vi "Set Values From HovaCAL Input.vi"(8 "error in (no error)":errorcluster caption="Fehler (Eingang, kein Fehler)") -> (0 "error out":errorcluster caption="Fehler (Ausgang)", 1 "HovaCAL Temperature":dbl[](array[numeric]) caption="Temp Setpoint" format="%.2f", 2 "SetPumpMode-Cluster":T4(array[cluster]) {"concentratio mode" items=["water", "reagent"]; "Reagent" items=["HCl", "HF", "NH3", "HG", "PPM", "ORGANIC"]}, 3 "Cluster.PumpModeGeneral":T8 caption="Pump Mode" {"dry mode" items=["wet", "dry"]; "control mode" items=["static", "pid"]}, 4 "Pump Concentrations-Cluster":T1[](array[typedef]) caption="Pump Setpoint", 5 "Set Values Cluster":T5(array[cluster]) caption="MFC Setpoints" {"output concentration setpoint" format="%.2f"; "input concentration setpoint" format="%.2f"}, 6 "Flow Input Cluster":cluster{"total flow setpoint":dbl} caption="Flow Setpoint" {"total flow setpoint" format="%.2f"}, 7 "Limits Cluster":cluster{"flow":dbl[], "temp":dbl[]} caption="Limits", 11 "SetPumpMode":cluster{"run":bool} caption="Pump")   [LabVIEW 2020, in "Linearisierung v2.lvlib" / "Gasteiler.lvlib" / "HovaCAL_Interface.lvlib" / "Kommunikation.lvlib"]
uses:
  Kommunikation.lvlib
  Controls/Pump Dry Mode.ctl
  Controls/Pump Control Mode.ctl
  Controls/Pump Concentration Mode.ctl
  Controls/Reagent.ctl
  Controls/Pump Concentration.ctl
  Aktion_FGV_HovaCAL_Interface_GetData.ctl
  Controls/Controls.lvlib
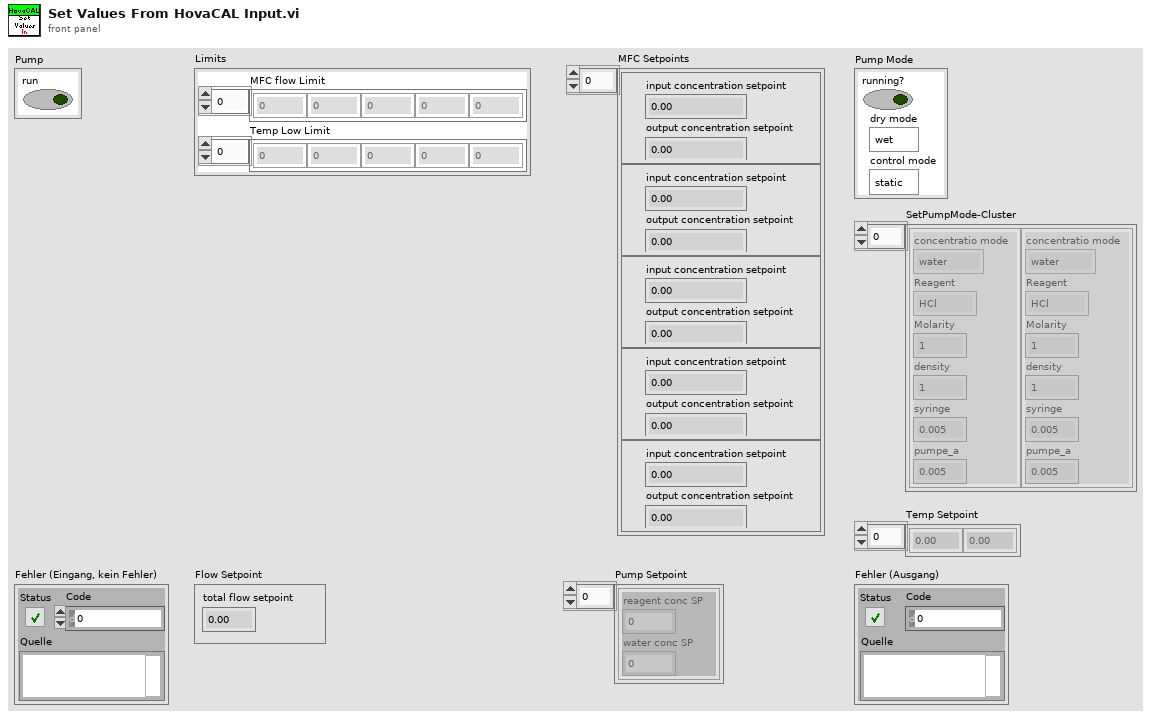
[diagram p1: front panel]
types:
  T1 = typedef "Linearisierung v2.lvlib/Gasteiler.lvlib/HovaCAL_Interface.lvlib/Controls.lvlib/Pump Concentration.ctl" = cluster{"reagent conc SP":dbl, "water conc SP":dbl}
  T2 = typedef "Linearisierung v2.lvlib/Gasteiler.lvlib/HovaCAL_Interface.lvlib/Controls.lvlib/Pump Concentration Mode.ctl" = i32
  T3 = typedef "Linearisierung v2.lvlib/Gasteiler.lvlib/HovaCAL_Interface.lvlib/Controls.lvlib/Reagent.ctl" = i32
  T4 = cluster{"concentratio mode":T2, "Reagent":T3, "Molarity":dbl, "density":dbl, "syringe":dbl, "pumpe_a":dbl}[]
  T5 = cluster{"input concentration setpoint":dbl, "output concentration setpoint":dbl}[]
  T6 = typedef "Linearisierung v2.lvlib/Gasteiler.lvlib/HovaCAL_Interface.lvlib/Controls.lvlib/Pump Dry Mode.ctl" = i32
  T7 = typedef "Linearisierung v2.lvlib/Gasteiler.lvlib/HovaCAL_Interface.lvlib/Controls.lvlib/Pump Control Mode.ctl" = u32
  T8 = cluster{"running?":bool, "dry mode":T6, "control mode":T7}
  T9 = cluster{"reagent conc SP":dbl, "water conc SP":dbl}
  T10 = cluster{"concentratio mode":T2, "Reagent":T3, "Molarity":dbl, "density":dbl, "syringe":dbl, "pumpe_a":dbl}
  T11 = cluster{"input concentration setpoint":dbl, "output concentration setpoint":dbl}
  T12 = typedef "Linearisierung v2.lvlib/Gasteiler.lvlib/HovaCAL_Interface.lvlib/Kommunikation.lvlib/Aktion_FGV_HovaCAL_Interface_GetData.ctl" = enum16{"lesen", "SystemInfo", "MFC Info", "actual Values", "Limits", "first contact", "reset after read"}
  T13 = cluster{"Input Concentrations (Ausgang)":cluster{"input concentration setpoint":dbl, "output concentration setpoint":dbl, "output concentration":dbl, "output concentration dry":dbl}[], "Cluster":cluster{"Temp Cluster":cluster{"temp SP":dbl, "temp":dbl, "humidity":dbl}[], "PumpModeGeneral-Cluster":cluster{"running?":bool, "dry mode":T6, "control mode":T7}, "PumpMode-Cluster":cluster{"Speed":dbl, "concentratio mode":T2, "Reagent":T3, "Molarity":dbl, "density":dbl, "syringe":dbl, "pumpe_a":dbl}[], "Pump Concentrations-Cluster":cluster{"reagent conc SP":dbl, "reagent conc":dbl, "reagent conc dry":dbl, "water conc SP":dbl, "water conc":dbl, "water conc dry":dbl}[], "Flow Output Cluster (Ausgang)":cluster{"total flow setpoint":dbl, "total flow":dbl}, "Pump MassFlow-Cluster":cluster{"reagent mf SP":dbl, "reagent mf":dbl, "water mf SP":dbl, "water mf":dbl, "water/reagent mf SP":dbl, "water/reagent mf":dbl}[], "MFC Flows-Cluster":cluster{"MFC  actual flow l/min":dbl, "MFC expected flow l/min":dbl}[]}}
  T14 = cluster{"input concentration setpoint":dbl, "output concentration setpoint":dbl, "output concentration":dbl, "output concentration dry":dbl}[]
  T15 = cluster{"temp SP":dbl, "temp":dbl, "humidity":dbl}[]
  T16 = cluster{"Speed":dbl, "concentratio mode":T2, "Reagent":T3, "Molarity":dbl, "density":dbl, "syringe":dbl, "pumpe_a":dbl}[]
  T17 = cluster{"reagent conc SP":dbl, "reagent conc":dbl, "reagent conc dry":dbl, "water conc SP":dbl, "water conc":dbl, "water conc dry":dbl}[]
  T18 = cluster{"total flow setpoint":dbl, "total flow":dbl}
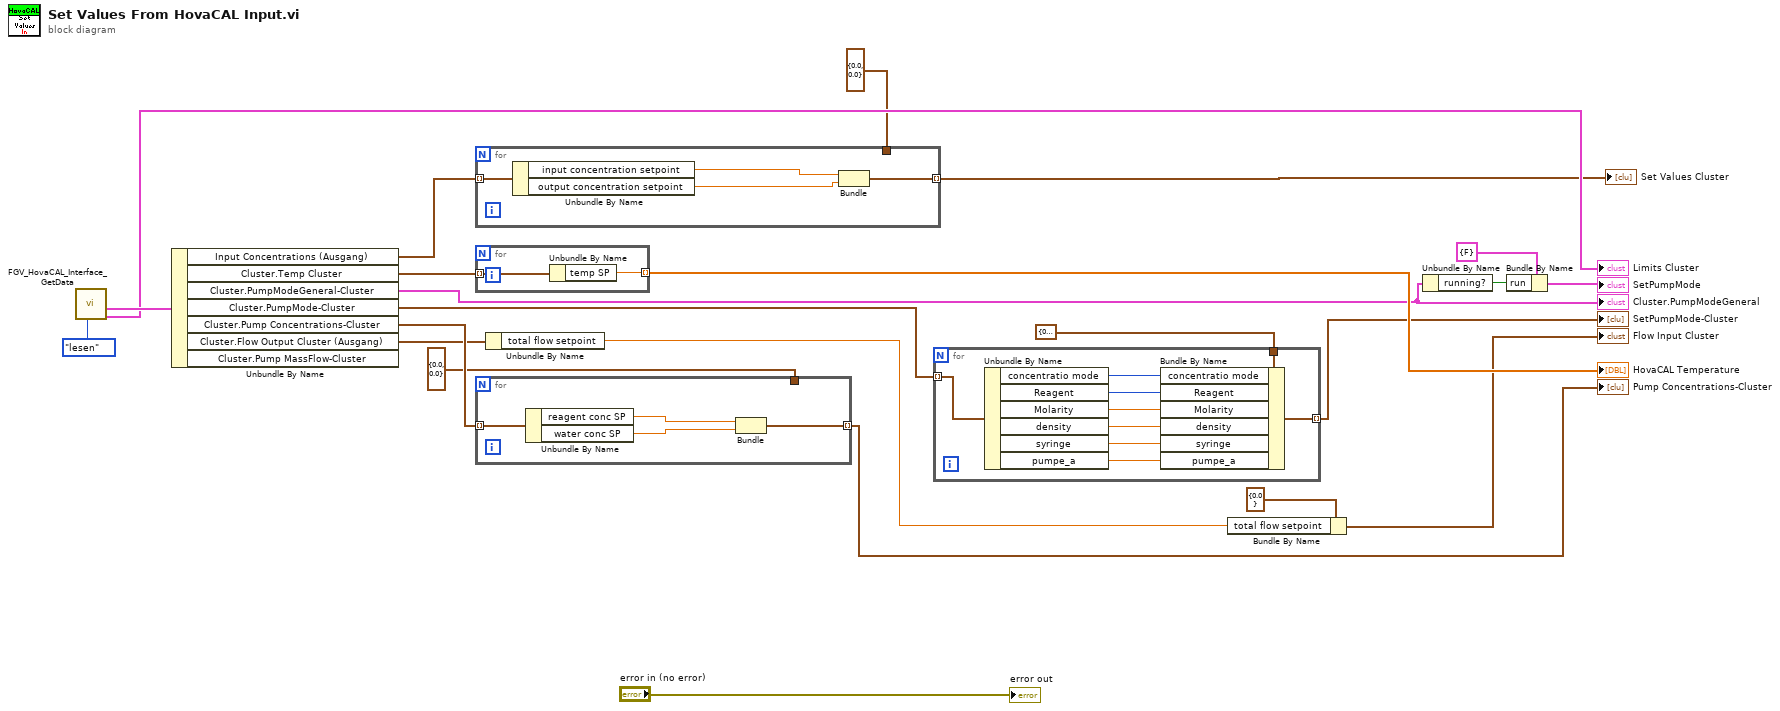
[diagram p0: block diagram]
diagram:
  n1 = call "FGV_HovaCAL_Interface_GetData.vi"("Aktion"=Aktion_FGV_HovaCAL_Interface_GetData."lesen") -> ("Limits Cluster out"=→"Limits Cluster":cluster{"flow":dbl[], "temp":dbl[]}, "actual Values Cluster out"=w22:T13)  [unwired: 6 in, 3 out]
  n2 = Unbundle By Name(w22) -> ("Input Concentrations (Ausgang)"=w21:T14, "Cluster.Temp Cluster"=w20:T15, "Cluster.PumpModeGeneral-Cluster"=w11:T8, "Cluster.PumpMode-Cluster"=w6:T16, "Cluster.Pump Concentrations-Cluster"=w19:T17, "Cluster.Flow Output Cluster (Ausgang)"=w17:T18)  [unwired: 1 out]
  "Cluster.PumpModeGeneral" <- w11
  n3 = for {
    tunnel: w21 -> [w27] mode=indexing
    tunnel: T11 {"input concentration setpoint"=0.0, "output concentration setpoint"=0.0} ("Set Values Cluster") -> [_]
    tunnel: [w24] -> w13 mode=indexing
    n4 = Unbundle By Name(w27) -> ("input concentration setpoint"=w26:dbl, "output concentration setpoint"=w25:dbl)
    n5 = Bundle("input concentration setpoint"=w26, "output concentration setpoint"=w25) -> (w24:T11)  [unwired: 1 in]
  }
  "Set Values Cluster" <- w13
  n6 = for {
    tunnel: w20 -> [w29] mode=indexing
    tunnel: [w28] -> w12 mode=indexing
    n7 = Unbundle By Name(w29) -> ("temp SP"=w28:dbl)
  }
  "HovaCAL Temperature" <- w12
  n8 = for {
    tunnel: w19 -> [w33] mode=indexing
    tunnel: T9 {"reagent conc SP"=0.0, "water conc SP"=0.0} ("Ausgangs-Cluster") -> [_]
    tunnel: [w31] -> w1 mode=indexing
    n9 = Unbundle By Name(w33) -> ("reagent conc SP"=w32:dbl, "water conc SP"=w30:dbl)
    n10 = Bundle("reagent conc SP"=w32, "water conc SP"=w30) -> (w31:T9)  [unwired: 1 in]
  }
  "Pump Concentrations-Cluster" <- w1
  n11 = Unbundle By Name(w17) -> ("total flow setpoint"=w16:dbl)
  n12 = for {
    tunnel: T10 {"concentratio mode"=0, "Reagent"=0, "Molarity"=1.0, "density"=1.0, "syringe"=0.005, "pumpe_a"=0.005} ("PumpMode-Cluster") -> [w42]
    tunnel: w6 -> [w41] mode=indexing
    tunnel: [w34] -> w5 mode=indexing
    n13 = Unbundle By Name(w41) -> ("concentratio mode"=w40:T2, "Reagent"=w39:T3, "Molarity"=w38:dbl, "density"=w37:dbl, "syringe"=w36:dbl, "pumpe_a"=w35:dbl)
    n14 = Bundle By Name(cluster=w42, "concentratio mode"=w40, "Reagent"=w39, "Molarity"=w38, "density"=w37, "syringe"=w36, "pumpe_a"=w35) -> (w34:T10)
  }
  "SetPumpMode-Cluster" <- w5
  n15 = Bundle By Name(cluster=cluster{"total flow setpoint":dbl} {"total flow setpoint"=0.0} ("Flow Input Cluster"), "total flow setpoint"=w16) -> (→"Flow Input Cluster":cluster{"total flow setpoint":dbl})
  n16 = Unbundle By Name(w11) -> ("running?"=w10:bool)
  n17 = Bundle By Name(cluster=cluster{"run":bool} {"run"=FALSE} ("SetPumpMode"), "run"=w10) -> (→"SetPumpMode":cluster{"run":bool})
  "error out" <- "error in (no error)"
